vi "NoCom(sous-VI).vi"(8 "entrée d'erreur (pas d'erreur)":errorcluster, 11 "Message Queue":refnum<queue>) -> (0 "error out":errorcluster, 3 "dup Message Queue":refnum<queue>)   [LabVIEW 2019]
uses:
  support/Message Queue/Message Cluster.ctl
  support/Message Queue/Enqueue Message (Single).vi
  support/Message Queue/Message Queue.lvlib
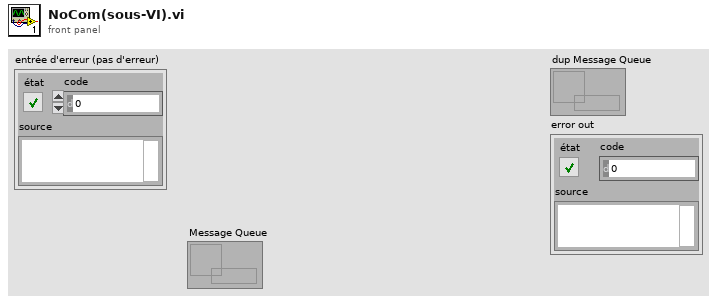
[diagram p1: front panel]
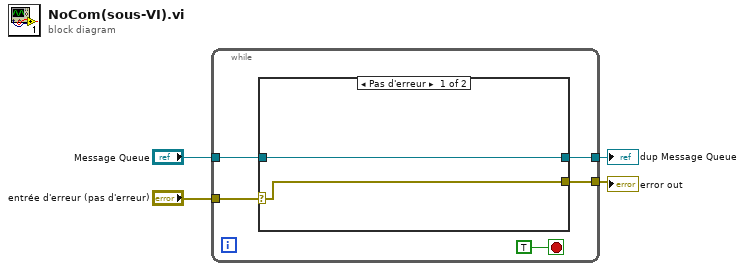
[diagram p0: block diagram]
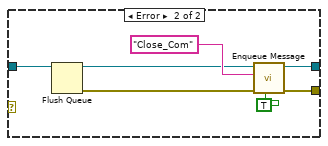
[diagram p2: hidden frame]
diagram:
  n1 = while {
    tunnel: "Message Queue" -> [w8]
    tunnel: [w7] -> w2
    tunnel: [w6] -> w3
    tunnel: "entrée d'erreur (pas d'erreur)" -> [w5]
    stop <- TRUE stop-if-true
    n2 = case shown="Pas d'erreur" w5 {
      selector: w5 -> [w10 _]
      tunnel: w8 -> [w11 w16]
      tunnel: [w10 w13] -> w7
      tunnel: [w11 w12] -> w6
      frame No Error {
      }
      frame Error {
        n3 = Flush Queue(queue=w16) -> (queue out=w15:refnum<queue>, error out=w14:errorcluster)  [unwired: 1 in, 1 out]
        n4 = call-poly "Enqueue Message.vi"("Priority Message? (F)"=TRUE, "error in (no error)"=w14, "Message"="Close_Com", "Message Queue"=w15) -> ("error out"=w13:errorcluster, "dup Message Queue"=w12:refnum<queue>)  [unwired: 6 in]
      }
    }
  }
  "dup Message Queue" <- w3
  "error out" <- w2
